vi "dtrsv - Solve Linear Eqs (Triangle, single) (DBL).vi"(4 "diagonal":T2 items=["Non-unit", "Unit"], 7 "operation A":T3 items=["Direct", "Conjugated & Transposed", "Transposed"], 8 "matrix A type":T1=3 items=["Lower Triangular"=2, "Upper Triangular"=3], 10 "x":dbl[](array[numeric]), 11 "A":T4) -> (0 "error":i32, 3 "dtrsv":dbl[](array[numeric]))   [LabVIEW 2014, in "NI_AALBLAS.lvlib"]
doc: "Solves the linear equation op(<B>A</B>)*<B>trsv</B> = <B>x</B> for <B>trsv</B>."
uses:
  NI_AALBLAS.lvlib
  RealMatrix.ctl
  LV_Transpose.ctl
  LV_Diag.ctl
  LV_UpLo.ctl
  Order.ctl
  Fucntion.ctl
  BLAS2 Utility(DBL).vi
  NI_Matrix.lvlib
panel:
  # "-1"
  # "dtrsv=op(A)  *x"
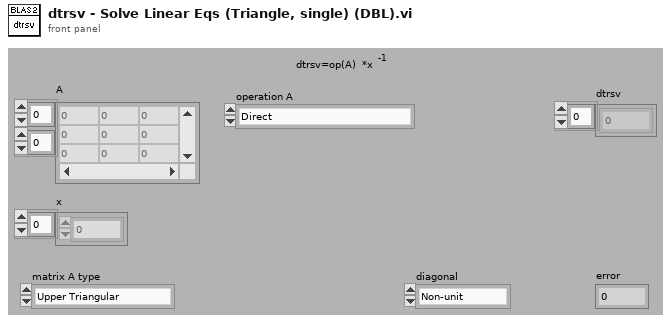
[diagram p1: front panel]
types:
  T1 = typedef "NI_AALBLAS.lvlib/LV_UpLo.ctl" = i32
  T2 = typedef "NI_AALBLAS.lvlib/LV_Diag.ctl" = i32
  T3 = typedef "NI_AALBLAS.lvlib/LV_Transpose.ctl" = i32
  T4 = typedef "NI_Matrix.lvlib/RealMatrix.ctl" = dbl[][]
  T5 = typedef "NI_AALBLAS.lvlib/Fucntion.ctl" = u16
  T6 = typedef "NI_AALBLAS.lvlib/Order.ctl" = i32
  T7 = typedef "NI_AALBLAS.lvlib/Diag.ctl" = i32
  T8 = typedef "NI_AALBLAS.lvlib/Operation_Transpose.ctl" = i32
  T9 = typedef "NI_AALBLAS.lvlib/UpLo.ctl" = i32
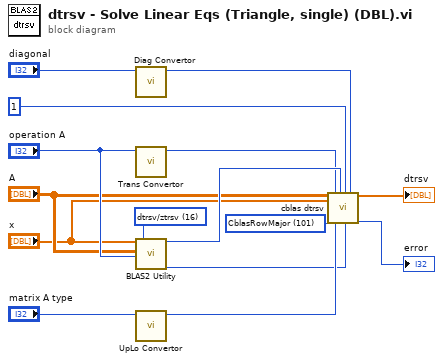
[diagram p0: block diagram]
diagram:
  w1 = T5 16 items=["ddot/zdotu/zdotc", "daxpy/zaxpy", "dnrm2/dznrm2", "dasum/dzasum", "dcopy/zcopy", "dswap/zswap", "drotm", "drot/zdrot", "idamax/izamax", "idamin/izamin", "dgemv/zgemv", "dsymv/zhemv", "dtrmv/ztrmv", "dsyr/zher", "dsyr2/zher2", "dger/zgeru/zgerc", "dtrsv/ztrsv", "dgemm/zgemm", "dsymm/zsymm/zhemm", "dtrmm/ztrmm", "dsyrk/zsyrk/zherk", "dsyr2k/zsyr2k/zher2k", "dtrsm/ztrsm"] ("function")
  w4 = T6 101 items=["CblasRowMajor"=101, "CblasColMajor"=102] ("order")
  n1 = call "Diag Convertor.vi"("diagonal"="diagonal") -> ("diag"=w9:T7)  [unwired: 10 out]
  n2 = call "Trans Convertor.vi"("operation"="operation A") -> ("trans"=w11:T8)  [unwired: 10 out]
  n3 = call-poly "BLAS2 Utility.vi"("x"="x", "A"="A", "operation A"="operation A", "function"=w1) -> ("lda"=w14:i32, "n"=w5:i32)  [unwired: 1 in, 13 out]
  n4 = call "UpLo Convertor.vi"("triangle matrix type"="matrix A type") -> ("uplo"=w12:T9)  [unwired: 10 out]
  n5 = call "cblas dtrsv.vi"("A"="A", "x"="x", "order"=w4, "transA"=w11, "uplo"=w12, "lda"=w14, "incx"=1, "n"=w5, "diag"=w9) -> ("dtrsv"=→"dtrsv":dbl[], "error"=→"error":i32)  [unwired: 9 out]
